vi "Test_PtByPtDiff.vi"() -> ()   [LabVIEW 2017]
uses:
  <vilib>/measure/NI_MABase.lvlib
panel:
  out "min difference":dbl
  out "max difference":dbl
  out "Waveform Chart":waveform(dbl)(graph)
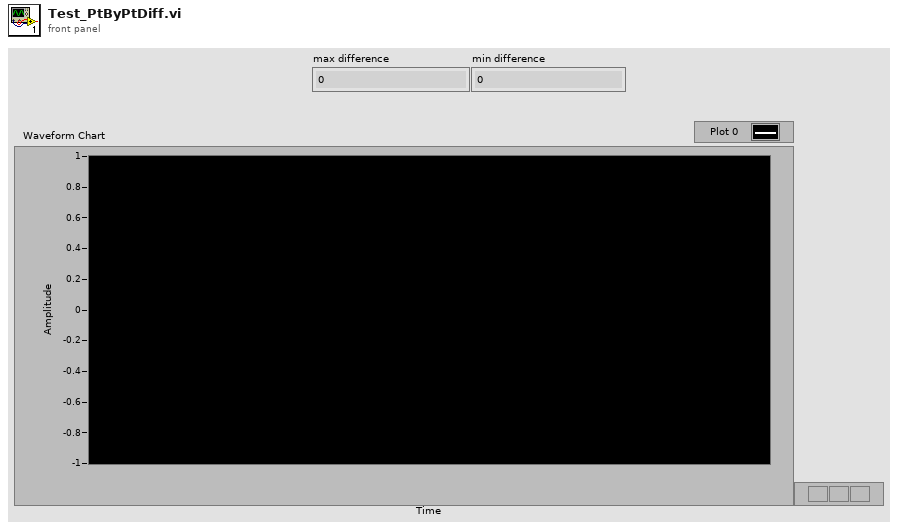
[diagram p1: front panel]
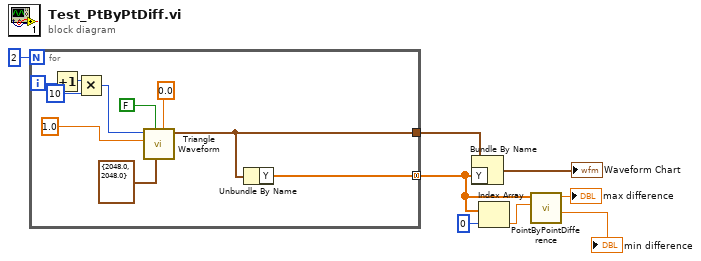
[diagram p0: block diagram]
diagram:
  n1 = for {
    N: 2 -> [_]
    tunnel: [w14] -> w8
    tunnel: [w13] -> w5 mode=concatenating
    i -> [w12]
    n2 = Increment(x=w12) -> (x+1=w11:i32)
    n3 = Multiply(x=w11, y=10) -> (x*y=w9:i32)
    n4 = call <vilib>:"Triangle Waveform.vi"("offset"=0.0, "sampling info"=cluster{"Fs":dbl, "#s":dbl} {"Fs"=2048.0, "#s"=2048.0}, "reset signal"=FALSE, "amplitude"=1.0, "frequency"=w9) -> ("signal out"=w14:waveform(dbl))  [unwired: 5 in, 1 out]
    n5 = Unbundle By Name(w14) -> ("Y"=w13:dbl[])
  }
  n6 = Bundle By Name(cluster=w8, "Y"=w5) -> (→"Waveform Chart":waveform(dbl))
  n7 = Index Array(array=w5, index=0) -> (element=w4:dbl)
  n8 = call <vilib>:"PointByPointDifference.vi"("initial condition"=w4, "array"=w5) -> ("min difference"=→"min difference":dbl, "max difference"=→"max difference":dbl)  [unwired: 7 in, 1 out]
